vi "GetLastImageName.vi"(1 "Path to folder":path) -> (0 "new path":path)   [LabVIEW 2009]
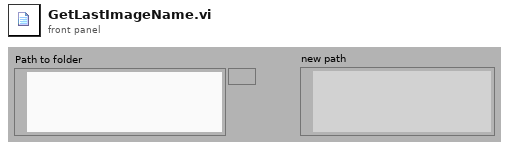
[diagram p1: front panel]
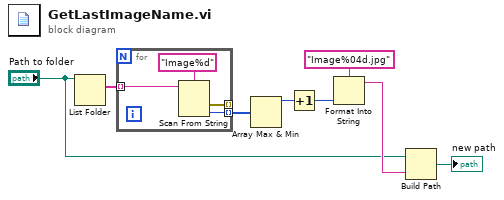
[diagram p0: block diagram]
diagram:
  n1 = List Folder(path="Path to folder") -> (filenames=w2:string[])  [unwired: 3 in, 3 out]
  n2 = for {
    tunnel: [w12] -> _ mode=indexing
    tunnel: w2 -> [w10] mode=indexing
    tunnel: [w9] -> w3 mode=indexing
    n3 = Scan From String(format string="Image%d", input string=w10) -> (error out=w12:errorcluster, output 1=w9:i32)  [unwired: 3 in, 2 out]
  }
  n4 = Array Max & Min(array=w3) -> (max value=w4:i32)  [unwired: 3 out]
  n5 = Increment(x=w4) -> (x+1=w1:i32)
  n6 = Format Into String(format string="Image%04d.jpg", w1) -> (resulting string=w7:string)  [unwired: 2 in, 1 out]
  n7 = Build Path(base path="Path to folder", name or relative path=w7) -> (appended path=→"new path":path)
